vi "Frecuencia.vi"(8 "error in (no error)":errorcluster, 10 "Frecuencia":dbl(slide) scale=0.0..10.0, 11 "Measurement in":refnum<class "Measurement.lvclass">) -> (0 "error out":errorcluster, 3 "Measurement out":refnum<class "Measurement.lvclass">)   [LabVIEW 2020, in "Measurement.lvlib" / "Measurement.lvclass"]
uses:
  Measurement.lvclass
  Measurement.lvclass/Measurement.ctl
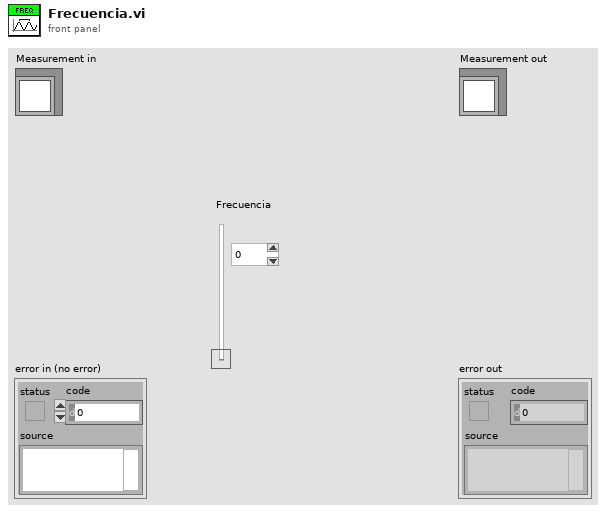
[diagram p1: front panel]
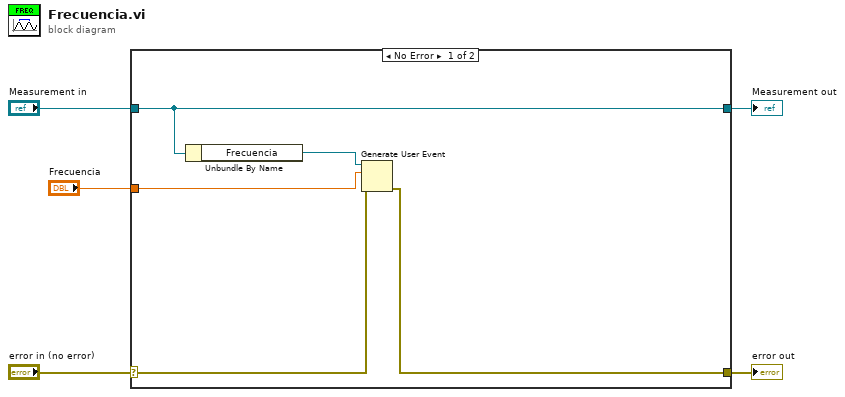
[diagram p0: block diagram]
diagram:
  n1 = case shown="No Error" "error in (no error)" {
    selector: "error in (no error)" -> [w7 w12]
    tunnel: [w6 w12] -> w4
    tunnel: [w10 w11] -> w2
    tunnel: "Measurement in" -> [w10 w11]
    tunnel: "Frecuencia" -> [w8 _]
    frame No Error {
      n2 = Unbundle By Name(w10) -> ("Frecuencia"=w9:refnum<user-event>)
      n3 = Generate User Event(user event=w9, event data cluster=w8, error in=w7) -> (error out=w6:errorcluster)  [unwired: 1 in, 1 out]
    }
    frame Error {
    }
  }
  "error out" <- w4
  "Measurement out" <- w2
